vi "Get Current Item.vi"(8 "error in (no error)":errorcluster caption="错误输入（无错误）", 11 "Iterator(Abstract) 输入":refnum<class "具体迭代器.lvclass"> caption="DNL_LabVIEW Object in") -> (0 "error out":errorcluster caption="错误输出", 2 "LabVIEW对象":refnum<class>, 3 "Iterator(Abstract) 输出":refnum<class "具体迭代器.lvclass"> caption="DNL_LabVIEW Object out")   [LabVIEW 2011, in "迭代器.lvlib" / "具体迭代器.lvclass"]
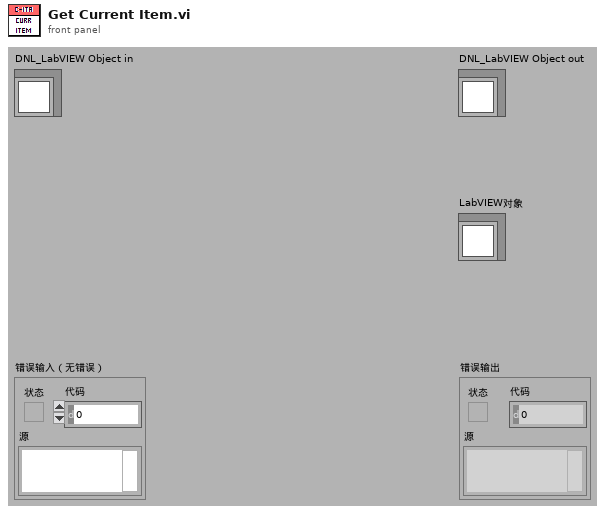
[diagram p1: front panel]
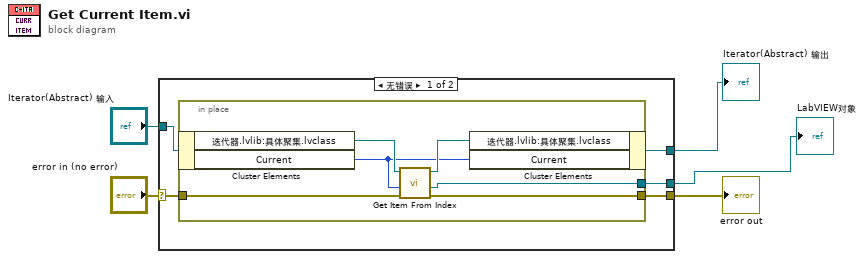
[diagram p0: block diagram]
diagram:
  n1 = case shown="无错误" "error in (no error)" {
    selector: "error in (no error)" -> [w7 w17]
    tunnel: [w6 w17] -> w4
    tunnel: "Iterator(Abstract) 输入" -> [w10 w18]
    tunnel: [w9 w18] -> w2
    tunnel: [w8 _] -> w1
    frame No Error {
      n2 = in-place {
        in-place-border: [w14] -> w8
        in-place-border: w7 -> [w12]
        in-place-border: [w11] -> w6
        n3 = in-place-cluster #1(w10) -> ("迭代器.lvlib:具体聚集.lvclass"=w16:refnum<class "具体聚集.lvclass">, "Current"=w13:i32)
        n4 = call "Get Item From Index.vi"("error in (no error)"=w12, "Index"=w13, "具体聚集 输入"=w16) -> ("error out"=w11:errorcluster, "迭代器.lvlib:雇员.lvclass"=w14:refnum<class "雇员.lvclass">, "具体聚集 输出"=w15:refnum<class "具体聚集.lvclass">)  [unwired: 6 in]
        n5 = in-place-cluster #1("迭代器.lvlib:具体聚集.lvclass"=w15, "Current"=w13) -> (w9:refnum<class "具体迭代器.lvclass">)
      }
    }
    frame Error {
    }
  }
  "error out" <- w4
  "Iterator(Abstract) 输出" <- w2
  "LabVIEW对象" <- w1
